vi "ValidPersonalNumber.vi"(10 "InputString":string) -> (2 "OutputString":string, 4 "Valid?":bool)   [LabVIEW 2022 SP3]
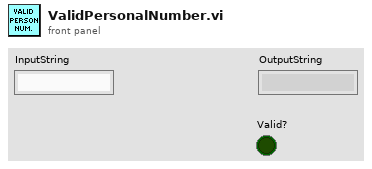
[diagram p1: front panel]
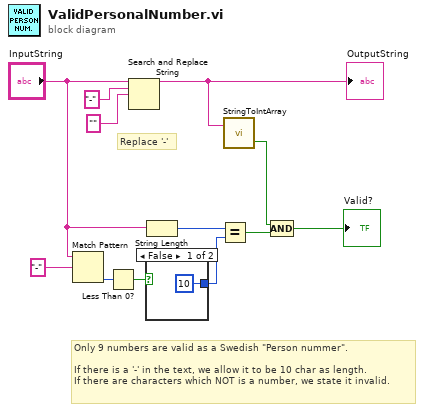
[diagram p0: block diagram]
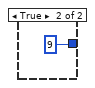
[diagram p2: hidden frame]
diagram:
  # "Replace '-'"
  # "Only 9 numbers are valid as a Swedish \"Person nummer\".\n\nIf there is a '-' in the text, we allow it to be 10 char as length.\nIf there are characters which NOT is a number, we state it invalid."
  n1 = Match Pattern(string="InputString", regular expression="-") -> (offset past match=w7:i32)  [unwired: 1 in, 3 out]
  n2 = Less Than 0?(x=w7) -> (x < 0?=w6:bool)
  n3 = Search and Replace String(input string="InputString", search string="-", replace string="" ("replace string (\"\")")) -> (result string=w2:string)  [unwired: 5 in, 3 out]
  "OutputString" <- w2
  n4 = case shown="False" w6 {
    tunnel: [10 ("y") 9 ("y")] -> w11
    frame False {
    }
    frame True {
    }
  }
  n5 = String Length(string="InputString") -> (length=w12:i32)
  n6 = Equal?(x=w12, y=w11) -> (x = y?=w9:bool)
  n7 = call "StringToIntArray.vi"("InputString"=w2) -> ("AllNumbers?"=w1:bool)  [unwired: 1 in, 1 out]
  n8 = Compound Arithmetic op=AND(w1, w9) -> (→"Valid?":bool)
